vi "bcd_to_7seg.vi"(9 "Number":u8) -> (1 "7-Seg. Array":bool[](array[boolean]))   [LabVIEW 2017]
doc: "This VI takes a U8 numeric and returns a boolean array decoded to display the numeric value on a 7 segment LED display.\n\nThis VI contains a single cycle timed loop. To use it within another single cycle timed loop, first remove the loop from within the VI.\n\n<b>Inputs:\nNumber</b> - Numeric value to decode. Values out of the range of 0-9 are treaded as don't care states, so the outputs for Number inputs outside of this range will not be useful.\n\n<b>\nOuputs:\n7-Seg. Array</b> - Array of boolen values reprosenting each of 7 segments on a 7 segment LED display. Index 0 corresponds to LED a, 1 corresponds to b, etc.. Please see the example for demonstration."
uses:
  <vilib>/Platform/TimedLoop/XDataNode/timing_clust.ctl
  <vilib>/Platform/TimedLoop/XDataNode/nitl_modes.ctl
  <vilib>/Platform/TimedLoop/XDataNode/wakeup.ctl
  <vilib>/Platform/TimedLoop/XDataNode/XDataNode.xnode
  <vilib>/Platform/TimedLoop/XDataNode/XDNodeRunTimeDep.lvlib
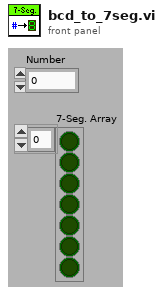
[diagram p1: front panel]
types:
  T1 = typedef "XDNodeRunTimeDep.lvlib/timing_clust.ctl" = cluster{"Expected End [f-1]":u64, "Actual End [f-1]":u64, "Finished Late? [f-1]":bool, "Expected End [i-1]":u64, "Actual End [i-1]":u64, "Finished Late? [i-1]":bool, "Expected Start [i]":u64, "Actual Start [i]":u64, "Expected Start [f]":u64, "Actual Start [f]":u64, "Source Name":string, "Structure Name":string, "Period":i64, "Deadline":i64, "Offset":i64, "Start":i64, "Priority":i32, "Timeout":i32, "Mode":T2, "Wakeup Reason":T3, "Error":errorcluster, "Source Type":string, "Secondary Source Type":string, "Global End Time":u64, "Global Start Time":u64, "Frame Duration":u64, "Iteration Duration":u64, "Assigned CPU":i32, "I/O Scan Engine Mode":u32}
  T2 = typedef "XDNodeRunTimeDep.lvlib/nitl_modes.ctl" = enum32{"No Change", "Process missed periods, maintain original phase", "Discard missed periods, maintain original phase", "Process missed periods, ignore original phase", "Discard missed periods, ignore original phase"}
  T3 = typedef "XDNodeRunTimeDep.lvlib/wakeup.ctl" = enum32{"Normal", "Aborted", "Asynchronous wakeup", "Timing source error", "Timed loop error", "Timeout"}
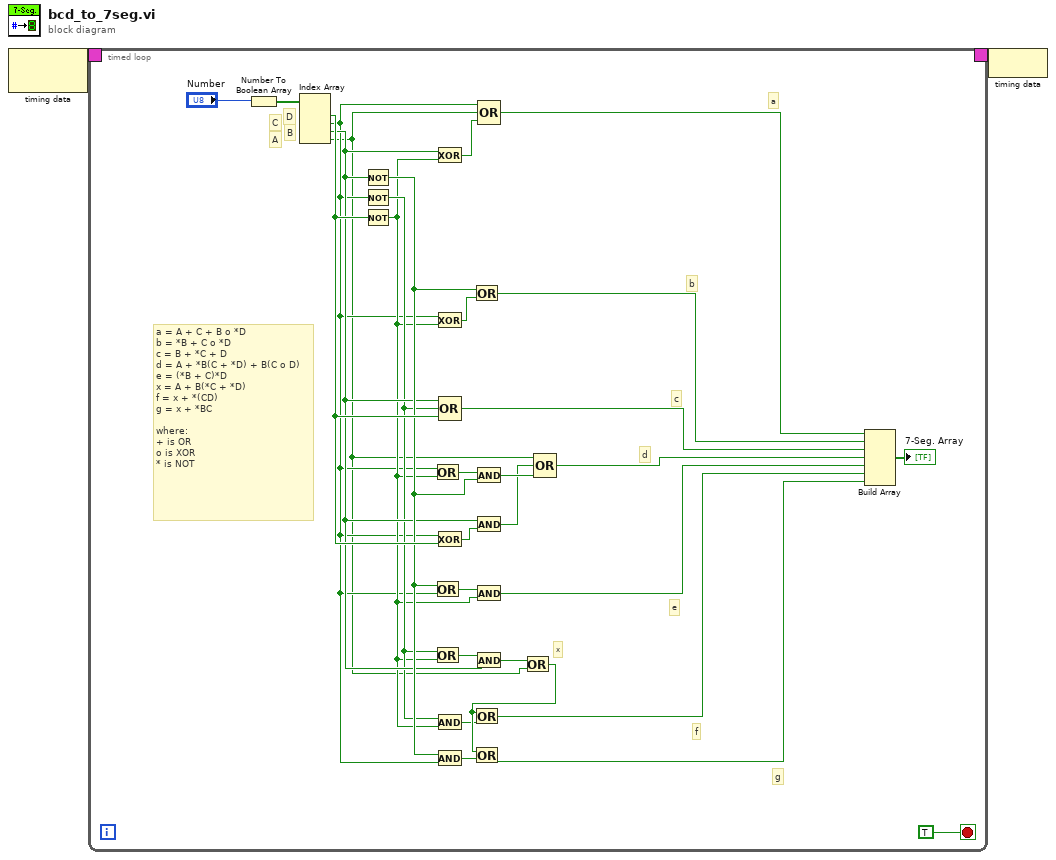
[diagram p0: block diagram]
diagram:
  n1 = node-c288() -> (w2:T1)  [unwired: 1 out]
  n2 = timed-loop {
    timing: w2 -> [_]
    timing-out: [_] -> w1
    stop <- TRUE stop-if-true
    # "g"
    # "f"
    # "e"
    # "d"
    # "c"
    # "b"
    # "a"
    # "a = A + C + B o *D\nb = *B + C o *D\nc = B + *C + D\nd = A + *B(C + *D) + B(C o D)\ne = (*B + C)*D\nx = A + B(*C + *D)\nf = x + *(CD)\ng = x + *BC\n\nwhere:\n+ is OR\no is XOR\n* is NOT"
    # "x"
    # "A"
    # "B"
    # "C"
    # "D"
    n3 = Number To Boolean Array(number="Number") -> (Boolean array=w15:bool[])
    n4 = Index Array(array=w15) -> (element #1=w22:bool, element #2=w6:bool, element #3=w20:bool, element #4=w5:bool)  [unwired: 4 in]
    n5 = Not(x=w20) -> (.not. x?=w21:bool)
    n6 = Not(x=w6) -> (.not. x?=w18:bool)
    n7 = Not(x=w22) -> (.not. x?=w17:bool)
    n8 = Or(x=w6, y=w17) -> (x .or. y?=w31:bool)
    n9 = Or(x=w21, y=w6) -> (x .or. y?=w27:bool)
    n10 = Or(x=w18, y=w17) -> (x .or. y?=w26:bool)
    n11 = Exclusive Or(1:w17, 2:w20) -> (0:w4:bool)
    n12 = Exclusive Or(1:w17, 2:w6) -> (0:w32:bool)
    n13 = Exclusive Or(1:w22, 2:w6) -> (0:w30:bool)
    n14 = And(x=w18, y=w17) -> (x .and. y?=w19:bool)
    n15 = And(x=w21, y=w6) -> (x .and. y?=w24:bool)
    n16 = Compound Arithmetic op=OR(w20, w18, w22) -> (w12:bool)
    n17 = Or(x=w21, y=w32) -> (x .or. y?=w13:bool)
    n18 = And(x=w31, y=w21) -> (x .and. y?=w29:bool)
    n19 = And(x=w20, y=w30) -> (x .and. y?=w28:bool)
    n20 = And(x=w27, y=w17) -> (x .and. y?=w10:bool)
    n21 = And(x=w26, y=w20) -> (x .and. y?=w25:bool)
    n22 = Compound Arithmetic op=OR(w6, w5, w4) -> (w14:bool)
    n23 = Or(x=w25, y=w5) -> (x .or. y?=w23:bool)
    n24 = Or(x=w23, y=w19) -> (x .or. y?=w9:bool)
    n25 = Or(x=w23, y=w24) -> (x .or. y?=w8:bool)
    n26 = Compound Arithmetic op=OR(w5, w29, w28) -> (w11:bool)
    n27 = Build Array(w14, w13, w12, w11, w10, w9, w8) -> (→"7-Seg. Array":bool[])
  }
  n28 = node-c288(w1) -> ()
